vi "spec_SetCenterWavelength.vi"(8 "error in (no error)":errorcluster, 10 "Center Wavelength":dbl, 11 "LightField Automation in":refnum<class "LightField Automation.lvclass">) -> (0 "error out":errorcluster, 3 "LightField Automation out":refnum<class "LightField Automation.lvclass">)   [LabVIEW 2018, in "LightField Automation.lvclass"]
uses:
  LightField Automation.lvclass
  C:/Users/xw9/Desktop/Turbulence program/SourceDistribution/PrincetonInstruments.LightFieldAddInSupportServices.dll
  PrincetonInstruments.LightFieldAddInSupportServices.dll
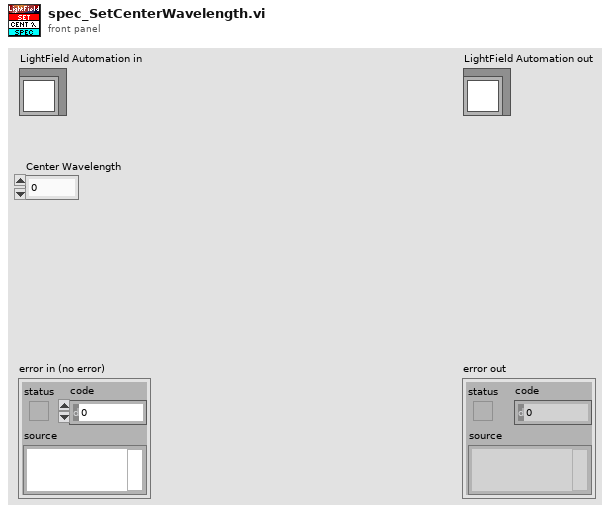
[diagram p1: front panel]
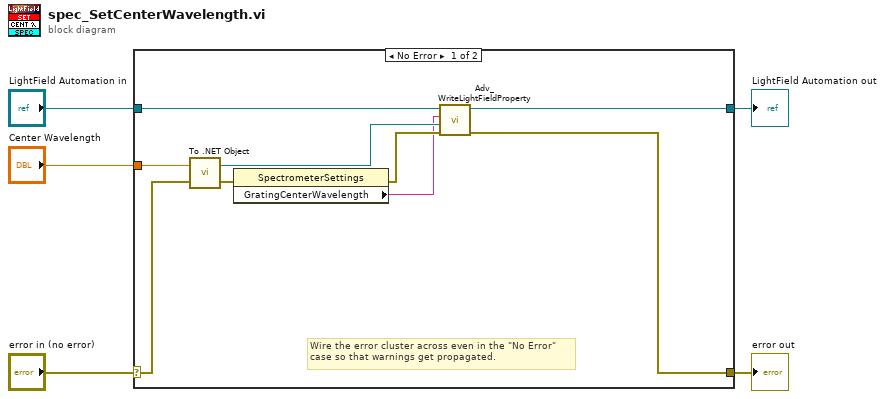
[diagram p0: block diagram]
diagram:
  n1 = case shown="No Error" "error in (no error)" {
    selector: "error in (no error)" -> [w13 w16]
    tunnel: [w8 w16] -> w4
    tunnel: [w7 w15] -> w2
    tunnel: "LightField Automation in" -> [w14 w15]
    tunnel: "Center Wavelength" -> [w6 _]
    frame No Error {
      # "Wire the error cluster across even in the \"No Error\"\ncase so that warnings get propagated."
      n2 = call "To .NET Object.vi"("error in (no error)"=w13, "anything"=w6) -> ("error out"=w11:errorcluster, ".NET object"=w12:refnum<k24>)
      n3 = property class="SpectrometerSettings"(error in=w11) -> (error out=w10:errorcluster, "GratingCenterWavelength"=w9:string)  [unwired: 1 in, 1 out]
      n4 = call "Adv_WriteLightFieldProperty.vi"("error in (no error)"=w10, "value"=w12, "setting"=w9, "LightField Automation in"=w14) -> ("error out"=w8:errorcluster, "LightField Automation out"=w7:refnum<class "LightField Automation.lvclass">)  [unwired: 6 in]
    }
    frame Error {
    }
  }
  "error out" <- w4
  "LightField Automation out" <- w2
